vi "sv_Buffer XY Data (N Ch).vi"(0 "XY signals":cluster{"X":dbl[], "Y":dbl[]}[](array[cluster]) {"X" format="%.2f"; "Y" format="%.2f"}, 2 "reset? (F)":bool, 11 "error in (no error)":errorcluster, 12 "buffer settings":T1 {"buffer mode" items=["Infinite length", "Last block data", "Custom"]}) -> (4 "buffered XY signals":cluster{"X":dbl[], "Y":dbl[]}[](array[cluster]) {"X" format="%.2f"; "Y" format="%.2f"}, 15 "error out":errorcluster)   [LabVIEW 2017]
doc: "Buffers the input signals and returns them in first-in first-out (FIFO) mode. The data type you wire to the <B>XY signal</B> input determines the polymorphic instance to use."
uses:
  <vilib>/addons/_NISVFA/_Shared subVIs/Controls/sv_Buffer XY Settings.ctl
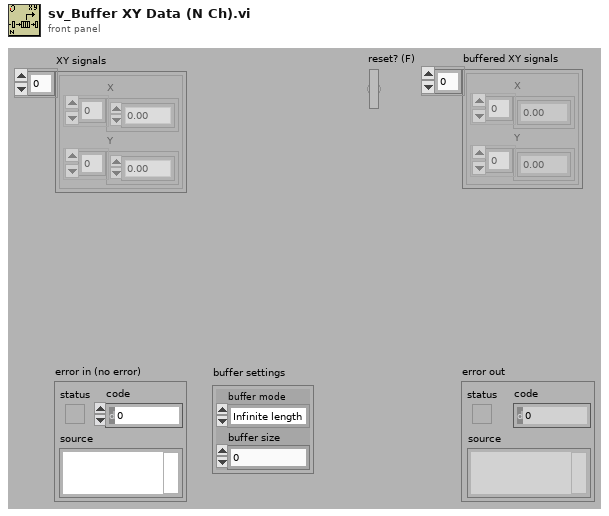
[diagram p1: front panel]
types:
  T1 = typedef "sv_Buffer XY Settings.ctl" = cluster{"buffer mode":u16, "buffer size":dbl}
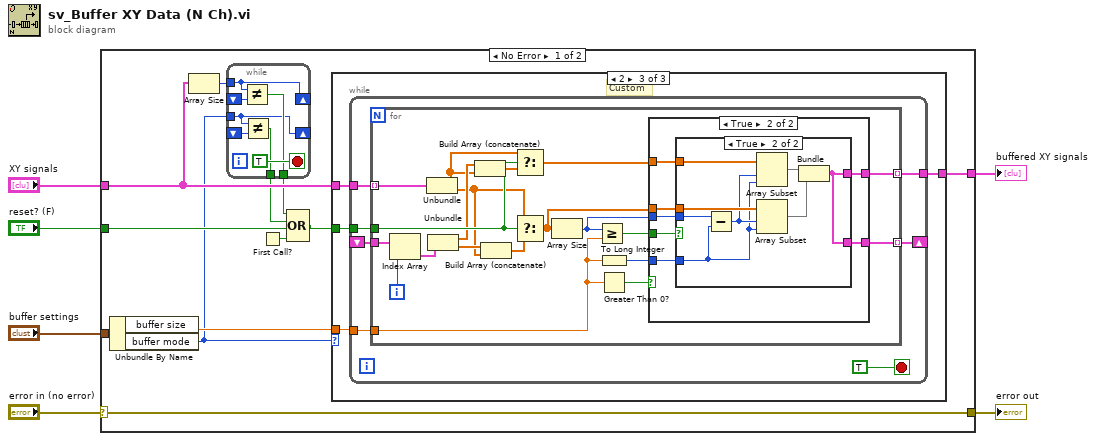
[diagram p0: block diagram]
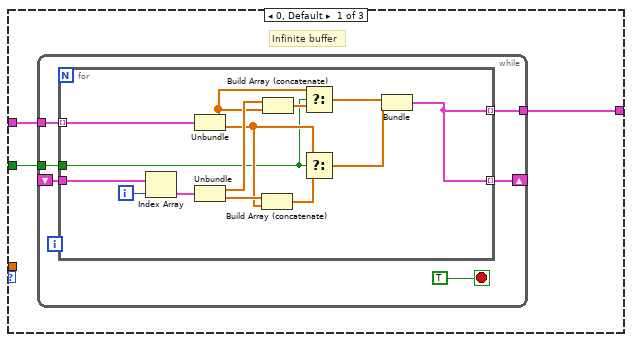
[diagram p2: hidden frame]
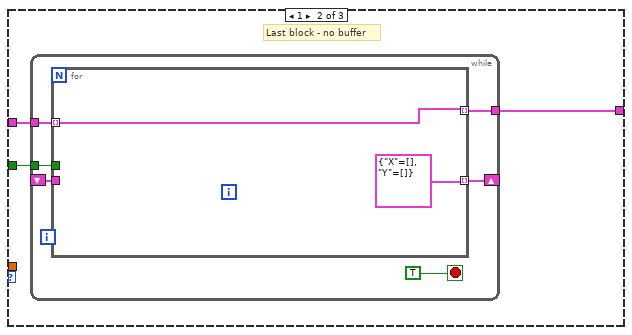
[diagram p3: hidden frame]
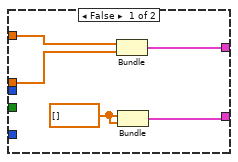
[diagram p4: hidden frame]
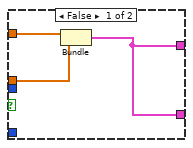
[diagram p5: hidden frame]
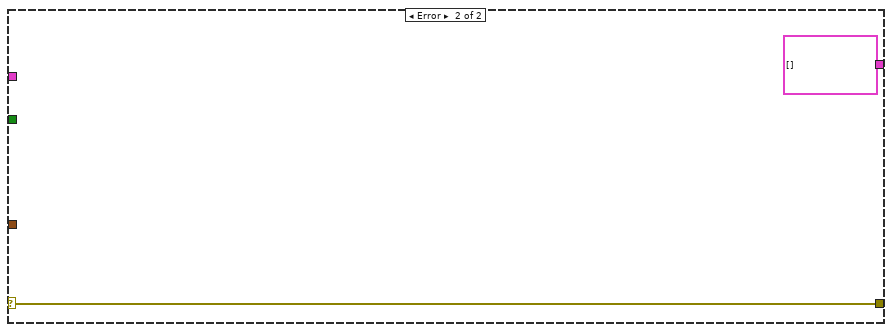
[diagram p6: hidden frame]
diagram:
  n1 = case shown="No Error" "error in (no error)" {
    selector: "error in (no error)" -> [w11 w115]
    tunnel: [w11 w115] -> w4
    tunnel: "buffer settings" -> [w18 _]
    tunnel: "XY signals" -> [w16 _]
    tunnel: "reset? (F)" -> [w14 _]
    tunnel: [w17 cluster{"X":dbl[], "Y":dbl[]}[] []] -> w3
    frame No Error {
      n2 = Unbundle By Name(w18) -> ("buffer size"=w10:dbl, "buffer mode"=w9:u16)
      n3 = Array Size(array=w16) -> (size(s)=w15:i32)
      n4 = while {
        tunnel: w15 -> [w24]
        shift-right: [w24] -> _
        shift-left: _ -> [w25]
        tunnel: [w22] -> w8
        tunnel: w9 -> [w19]
        shift-right: [w19] -> _
        shift-left: _ -> [w21]
        tunnel: [w20] -> w7
        stop <- TRUE stop-if-true
        n5 = Not Equal?(x=w24, y=w25) -> (x != y?=w22:bool)
        n6 = Not Equal?(x=w19, y=w21) -> (x != y?=w20:bool)
      }
      n7 = First Call?() -> (First Call?: T/F=w13:bool)
      n8 = Compound Arithmetic op=OR(w8, w7, w14, w13) -> (w12:bool)
      n9 = case shown="2" w9 {
        tunnel: w10 -> [_ _ w61]
        tunnel: w16 -> [w27 w50 w63]
        tunnel: w12 -> [w26 w49 w62]
        tunnel: [w28 w51 w60] -> w17
        frame 0, Default {
          # "Infinite buffer"
          n10 = while {
            tunnel: [w34] -> w28
            tunnel: w27 -> [w30]
            shift-right: [w33] -> _
            shift-left: _ -> [w31]
            tunnel: w26 -> [w29]
            stop <- TRUE stop-if-true
            n11 = for {
              tunnel: [w35] -> w34 mode=indexing
              tunnel: [w35] -> w33 mode=indexing
              tunnel: w31 -> [w40]
              tunnel: w30 -> [w42] mode=indexing
              tunnel: w29 -> [w37]
              i -> [w38]
              n12 = Index Array(array=w40, index=w38) -> (element=w39:cluster{"X":dbl[], "Y":dbl[]})
              n13 = Unbundle(w42) -> ("X"=w47:dbl[], "Y"=w44:dbl[])
              n14 = Unbundle(w39) -> ("X"=w48:dbl[], "Y"=w45:dbl[])
              n15 = Build Array (concatenate)(w45, w44) -> (w43:dbl[])
              n16 = Build Array (concatenate)(w48, w47) -> (w46:dbl[])
              n17 = Select(t=w47, s=w37, f=w46) -> (s? t:f=w36:dbl[])
              n18 = Select(t=w44, s=w37, f=w43) -> (s? t:f=w41:dbl[])
              n19 = Bundle("X"=w36, "Y"=w41) -> (w35:cluster{"X":dbl[], "Y":dbl[]})  [unwired: 1 in]
            }
          }
        }
        frame 1 {
          # "Last block - no buffer"
          n20 = while {
            tunnel: [w57] -> w51
            tunnel: w50 -> [w53]
            shift-right: [w56] -> _
            shift-left: _ -> [w54]
            tunnel: w49 -> [w52]
            stop <- TRUE stop-if-true
            n21 = for {
              tunnel: [w58] -> w57 mode=indexing
              tunnel: [cluster{"X":dbl[], "Y":dbl[]} {"X"=[], "Y"=[]} ("output cluster")] -> w56 mode=indexing
              tunnel: w54 -> [_]
              tunnel: w53 -> [w58] mode=indexing
              tunnel: w52 -> [_]
            }
          }
        }
        frame 2 {
          # "Custom"
          n22 = while {
            tunnel: w63 -> [w70]
            shift-right: [w66] -> _
            shift-left: _ -> [w64]
            tunnel: w62 -> [w67]
            tunnel: w61 -> [w68]
            tunnel: [w65] -> w60
            stop <- TRUE stop-if-true
            n23 = for {
              tunnel: w70 -> [w90] mode=indexing
              tunnel: w68 -> [w71]
              tunnel: w67 -> [w86]
              tunnel: [w84] -> w66 mode=indexing
              tunnel: [w83] -> w65 mode=indexing
              tunnel: w64 -> [w75]
              i -> [w74]
              n24 = Index Array(array=w75, index=w74) -> (element=w73:cluster{"X":dbl[], "Y":dbl[]})
              n25 = Unbundle(w90) -> ("X"=w80:dbl[], "Y"=w77:dbl[])
              n26 = Unbundle(w73) -> ("X"=w81:dbl[], "Y"=w78:dbl[])
              n27 = Build Array (concatenate)(w81, w80) -> (w79:dbl[])
              n28 = Build Array (concatenate)(w78, w77) -> (w76:dbl[])
              n29 = Select(t=w80, s=w86, f=w79) -> (s? t:f=w85:dbl[])
              n30 = Select(t=w77, s=w86, f=w76) -> (s? t:f=w89:dbl[])
              n31 = Array Size(array=w89) -> (size(s)=w88:i32)
              n32 = Greater Or Equal?(x=w88, y=w71) -> (x >= y?=w82:bool)
              n33 = To Long Integer(number=w71) -> (32bit integer=w87:i32)
              n34 = Greater Than 0?(x=w71) -> (x > 0?=w72:bool)
              n35 = case shown="True" w72 {
                tunnel: w89 -> [w94 w102]
                tunnel: w88 -> [_ w101]
                tunnel: w87 -> [_ w100]
                tunnel: w85 -> [w95 w99]
                tunnel: [w91 w98] -> w84
                tunnel: [w93 w97] -> w83
                tunnel: w82 -> [_ w96]
                frame False {
                  w92 = dbl[] [] ("Y")
                  n36 = Bundle("X"=w95, "Y"=w94) -> (w93:cluster{"X":dbl[], "Y":dbl[]})  [unwired: 1 in]
                  n37 = Bundle("Y"=w92, "Y"=w92) -> (w91:cluster{"Y":dbl[], "Y":dbl[]})  [unwired: 1 in]
                }
                frame True {
                  n38 = case shown="True" w96 {
                    tunnel: w102 -> [w104 w113]
                    tunnel: w100 -> [_ w109]
                    tunnel: w101 -> [_ w112]
                    tunnel: w99 -> [w105 w111]
                    tunnel: [w103 w106] -> w98
                    tunnel: [w103 w106] -> w97
                    frame False {
                      n39 = Bundle("X"=w105, "Y"=w104) -> (w103:cluster{"X":dbl[], "Y":dbl[]})  [unwired: 1 in]
                    }
                    frame True {
                      n40 = Subtract(x=w112, y=w109) -> (x-y=w110:i32)
                      n41 = Array Subset(array=w111, index=w110, length=w109) -> (w108:dbl[])
                      n42 = Array Subset(array=w113, index=w110, length=w109) -> (w107:dbl[])
                      n43 = Bundle(w108, w107) -> (w106:cluster{dbl[], dbl[]})  [unwired: 1 in]
                    }
                  }
                }
              }
            }
          }
        }
      }
    }
    frame Error {
    }
  }
  "error out" <- w4
  "buffered XY signals" <- w3
